vi "ITX to LV 2.1 1D.vi"(0 "file (use dialog)":path=path "P:/sample/GaAs/GaAs quantum dots/2008/PL Map/A1 735/060731ASBA_A1_6.0.itx") -> (3 "1D arrays":dbl[][](array[numeric]), 4 "wave names":string[](array[string]), 5 "Notes":string)   [LabVIEW 2013]
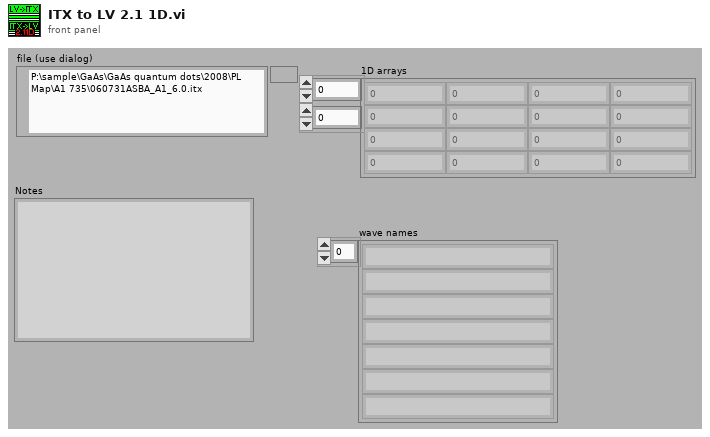
[diagram p1: front panel]
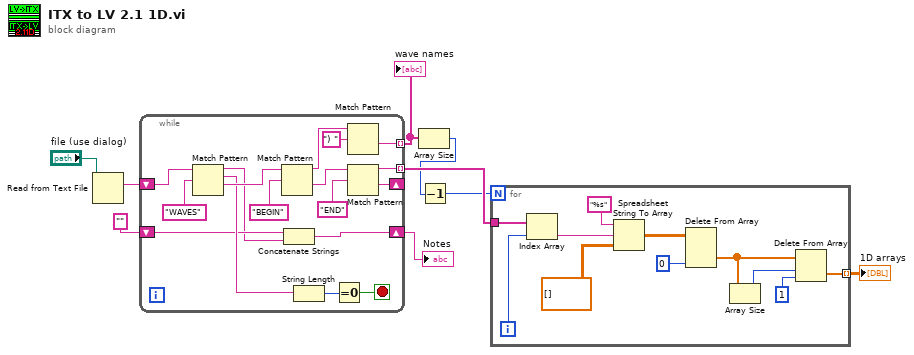
[diagram p0: block diagram]
diagram:
  n1 = Read from Text File(file (use dialog)="file (use dialog)") -> (text=w9:string)  [unwired: 2 in, 4 out]
  n2 = while {
    tunnel: [w10] -> w6 mode=indexing
    shift-right: [w24] -> _
    shift-left: w9 -> [w12]
    tunnel: [w20] -> w4 mode=indexing
    shift-right: [w15] -> w5
    shift-left: "" ("regular expression") -> [w14]
    stop <- w21 stop-if-true
    n3 = Match Pattern(string=w12, regular expression="WAVES") -> (before substring=w13:string, match substring=w23:string, after substring=w26:string)  [unwired: 2 out]
    n4 = Match Pattern(string=w26, regular expression="BEGIN" ("regular expression 2")) -> (before substring=w11:string, after substring=w25:string)  [unwired: 3 out]
    n5 = Concatenate Strings(w14, w13) -> (w15:string)
    n6 = String Length(string=w23) -> (length=w22:i32)
    n7 = Equal To 0?(x=w22) -> (x = 0?=w21:bool)
    n8 = Match Pattern(string=w11, regular expression=") ") -> (after substring=w20:string)  [unwired: 4 out]
    n9 = Match Pattern(string=w25, regular expression="END" ("regular expression 3")) -> (before substring=w10:string, after substring=w24:string)  [unwired: 3 out]
  }
  "wave names" <- w4
  "Notes" <- w5
  n10 = Array Size(array=w4) -> (size(s)=w3:i32)
  n11 = Decrement(x=w3) -> (x-1=w1:i32)
  n12 = for {
    N: w1 -> [_]
    tunnel: [w35] -> w8 mode=indexing
    tunnel: w6 -> [w31]
    i -> [w27]
    n13 = Index Array(array=w31, index=w27) -> (element=w30:string)
    n14 = Spreadsheet String To Array(format string="%s", spreadsheet string=w30, array type (2D Dbl)=dbl[][] []) -> (array=w36:dbl[][])  [unwired: 1 out]
    n15 = Delete From Array(array=w36, index (col)=0 ("disabled index (col)")) -> (deleted portion=w34:dbl[])  [unwired: 2 in, 1 out]
    n16 = Array Size(array=w34) -> (size(s)=w33:i32)
    n17 = Delete From Array(array=w34, length=w33, index=1) -> (deleted portion=w35:dbl[])  [unwired: 1 out]
  }
  "1D arrays" <- w8
